vi "Dryer_DSM_CMD.vi"(10 "Command":T1=2 items=["CMD_Eval_Mode_Entry_CC1", "CMD_Eval_Mode_Entry_CC2", "CMD_Eval_Mode_Continue", "CMD_Send_DIAG_Info", "CMD_Enable_Debug_Log ", "CMD_Disable_Debug_Log ", "CMD_Send_Log_Data", "CMD_Stop", "RQST_Version"]) -> (2 "CMD Array":u8[](array[numeric])=[115, 0] format="%02x")   [LabVIEW 2012]
doc: "Given the command array, this VI will look up the associated Hex numaric and output that value"
uses:
  Dryer Commands.ctl
panel:
  in  "Commands":cluster{"String":string, "CMD Array":u8[]}[](array[cluster])=[{"String"="CMD_Eval_Mode_Entry_CC1", "CMD Array"=[112, 1]}, {"String"="CMD_Eval_Mode_Entry_CC2", "CMD Array"=[112, 2]}, {"String"="CMD_Eval_Mode_Continue", "CMD Array"=[113]}, {"String"="CMD_Send_DIAG_Info", "CMD Array"=[114]}, {"String"="CMD_Enable_Debug_Log ", "CMD Array"=[115, 1]}, {"String"="CMD_Disable_Debug_Log ", "CMD Array"=[115, 0]}, {"String"="CMD_Send_Log_Data", "CMD Array"=[116]}, {"String"="CMD_Stop", "CMD Array"=[118]}, {"String"="RQST_Version", "CMD Array"=[1]}] {"CMD Array" format="%02x"}
  out "Data Array":string[][](array[string])=[["CMD_Eval_Mode_Entry_CC1", "0x70", "0x01"], ["CMD_Eval_Mode_Entry_CC2", "0x70", "0x02"], ["CMD_Eval_Mode_Continue", "0x71", "N/A"], ["CMD_Send_DIAG_Info", "0x72", "N/A"], ["CMD_Enable_Debug_Log ", "0x73", "0x01"], ["CMD_Disable_Debug_Log ", "0x73", "0x00"], ["CMD_Send_Log_Data", "0x74", "N/A"]]
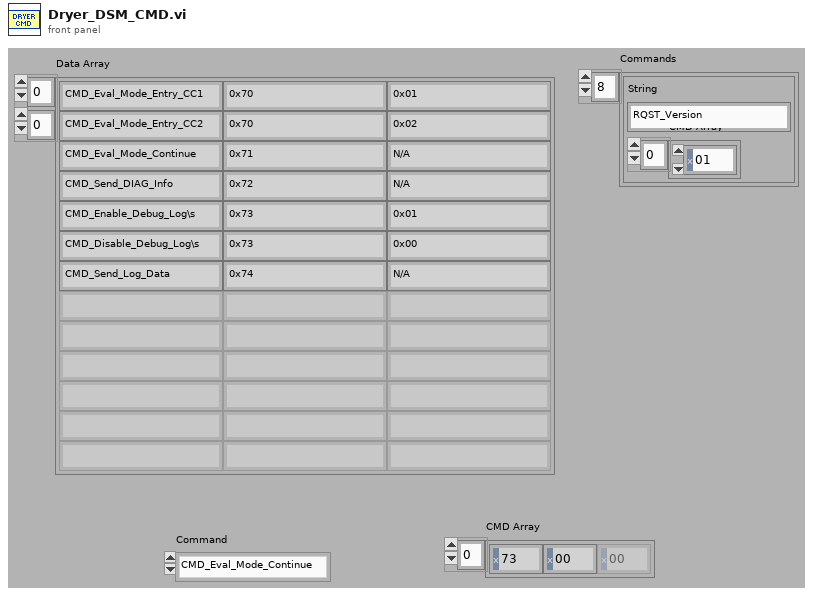
[diagram p1: front panel]
types:
  T1 = typedef "Dryer Commands.ctl" = u8
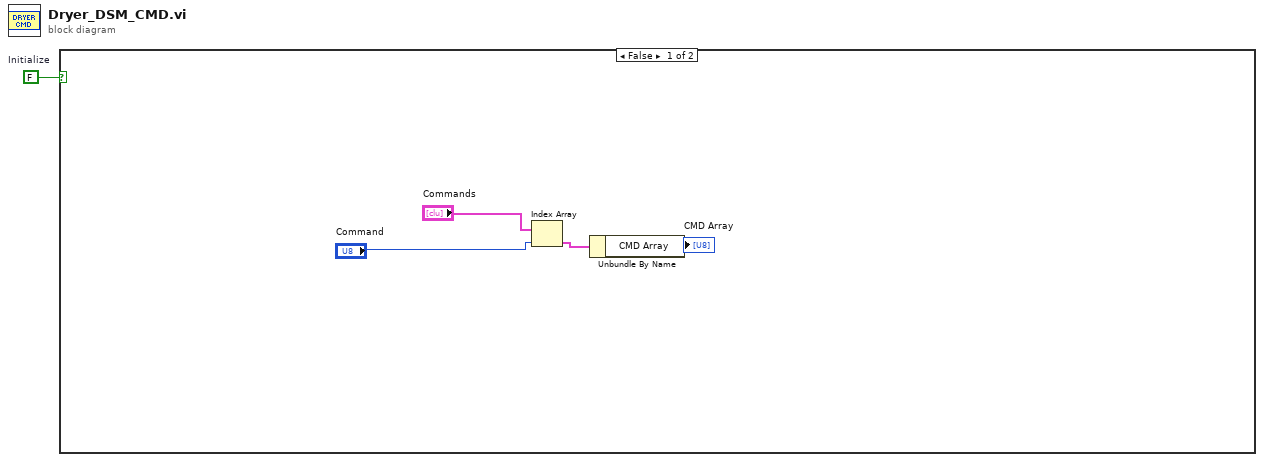
[diagram p0: block diagram]
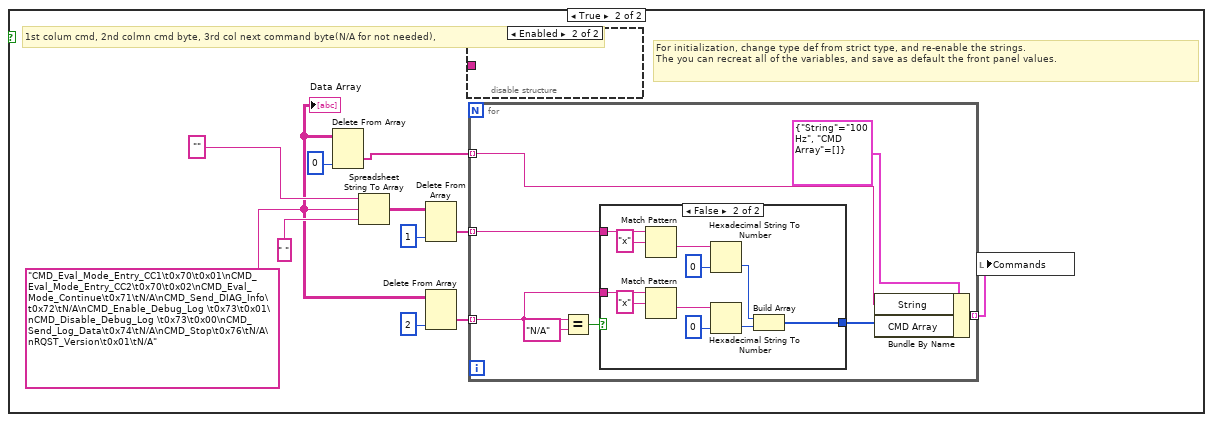
[diagram p2: hidden frame]
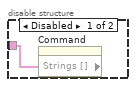
[diagram p3: hidden frame]
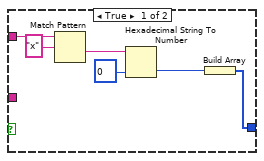
[diagram p4: hidden frame]
diagram:
  w1 = FALSE  # Initialize
  n1 = case shown="False" w1 {
    frame False {
      n2 = Index Array(array="Commands", index="Command") -> (element=w4:cluster{"String":string, "CMD Array":u8[]})
      n3 = Unbundle By Name(w4) -> ("CMD Array"=→"CMD Array":u8[])
    }
    frame True {
      # "For initialization, change type def from strict type, and re-enable the strings.\nThe you can recreat all of the variables, and save as default the front panel values."
      # "1st colum cmd, 2nd colmn cmd byte, 3rd col next command byte(N/A for not needed),"
      n4 = Spreadsheet String To Array(format string="", spreadsheet string="CMD_Eval_Mode_Entry_CC1\t0x70\t0x01\nCMD_Eval_Mode_Entry_CC2\t0x70\t0x02\nCMD_Eval_Mode_Continue\t0x71\tN/A\nCMD_Send_DIAG_Info\t0x72\tN/A\nCMD_Enable_Debug_Log \t0x73\t0x01\nCMD_Disable_Debug_Log \t0x73\t0x00\nCMD_Send_Log_Data\t0x74\tN/A\nCMD_Stop\t0x76\tN/A\nRQST_Version\t0x01\tN/A", array type (2D Dbl)=" " ("delimiter (Tab)")) -> (array=w9:string[][])  [unwired: 1 in]
      "Data Array" <- w9
      n5 = Delete From Array(array=w9, index (col)=0 ("disabled index (col)")) -> (deleted portion=w6:string[])  [unwired: 2 in, 1 out]
      n6 = Delete From Array(array=w9, index (col)=1 ("disabled index (col)")) -> (deleted portion=w11:string[])  [unwired: 2 in, 1 out]
      n7 = Delete From Array(array=w9, index (col)=2 ("disabled index (col)")) -> (deleted portion=w8:string[])  [unwired: 2 in, 1 out]
      n8 = disable-structure shown="Enabled" {
        disable-tunnel: [w17 _] -> _
        frame Disabled {
          n9 = property on="Command" class="Ring (strict)"() -> ("Strings []"=w17:string[])  [unwired: 2 in, 2 out]
        }
        frame Enabled {
        }
      }
      n10 = for {
        tunnel: w6 -> [w24] mode=indexing
        tunnel: w11 -> [w23] mode=indexing
        tunnel: [w22] -> w7 mode=indexing
        tunnel: w8 -> [w18] mode=indexing
        n11 = Equal?(x=w18, y="N/A") -> (x = y?=w19:bool)
        n12 = case shown="False" w19 {
          tunnel: w23 -> [w31 w42]
          tunnel: [w26 w38] -> w21
          tunnel: w18 -> [_ w36]
          frame True {
            n13 = Match Pattern(string=w31, regular expression="x") -> (after substring=w29:string)  [unwired: 1 in, 3 out]
            n14 = Hexadecimal String To Number(string=w29, default (0uL)=u8 0 ("default (0 U32)")) -> (number=w27:u8)  [unwired: 1 in, 1 out]
            n15 = Build Array(w27) -> (w26:u8[])
          }
          frame False {
            n16 = Match Pattern(string=w42, regular expression="x") -> (after substring=w40:string)  [unwired: 1 in, 3 out]
            n17 = Match Pattern(string=w36, regular expression="x") -> (after substring=w33:string)  [unwired: 1 in, 3 out]
            n18 = Hexadecimal String To Number(string=w40, default (0uL)=u8 0 ("default (0 U32)")) -> (number=w39:u8)  [unwired: 1 in, 1 out]
            n19 = Hexadecimal String To Number(string=w33, default (0uL)=u8 0 ("default (0 U32)")) -> (number=w32:u8)  [unwired: 1 in, 1 out]
            n20 = Build Array(w39, w32) -> (w38:u8[])
          }
        }
        n21 = Bundle By Name(cluster=cluster{"String":string, "CMD Array":u8[]} {"String"="100 Hz", "CMD Array"=[]}, "String"=w24, "CMD Array"=w21) -> (w22:cluster{"String":string, "CMD Array":u8[]})
      }
      n22 = local write "Commands"(w7) -> ()
    }
  }
